vi "what_do_you_want.vi"() -> (0 "Next state":T1(ring), 1 "Leave":bool)   [LabVIEW 2014]
panel:
  in  "Cluster":T2
  # "You have pressed the cancel buttom.\nWhat do you want to do now?\n1.Choose seats again.\n2.Select another movie.\n3.Leave the movie booking system"
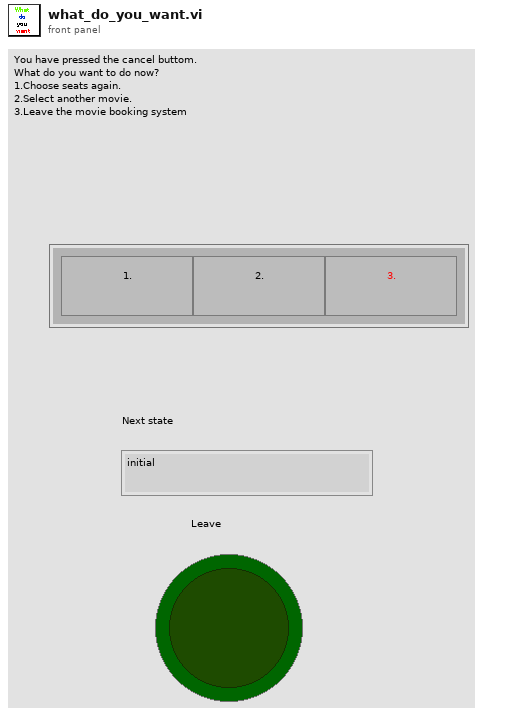
[diagram p1: front panel]
types:
  T1 = enum16{"initial", "start", "member?", "register?", "member login", "member register", "choose movie", "how many seat?", "check", "end"}
  T2 = cluster{"OK Button":bool, "OK Button 2":bool, "stop":bool}
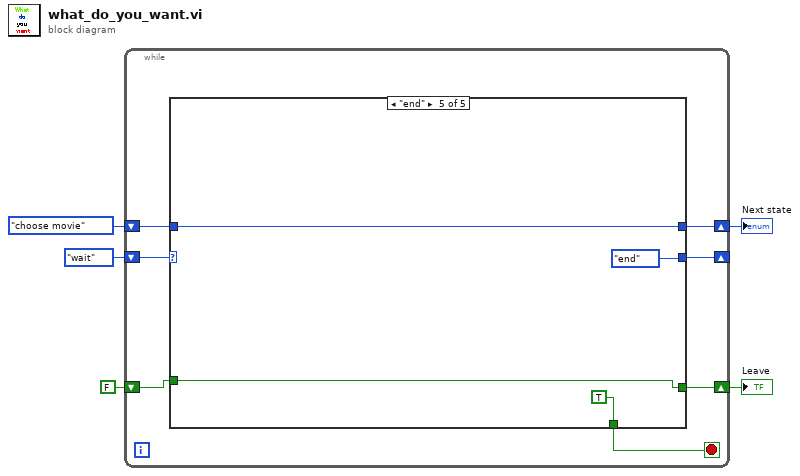
[diagram p0: block diagram]
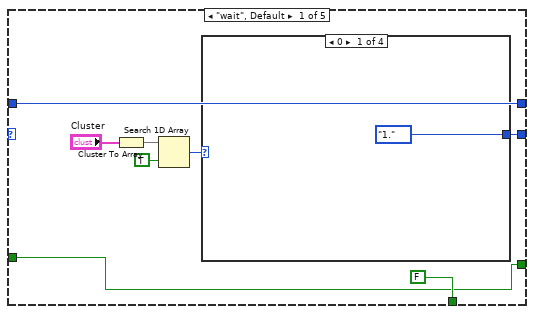
[diagram p2: hidden frame]
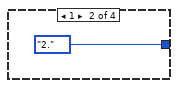
[diagram p3: hidden frame]
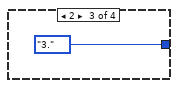
[diagram p4: hidden frame]
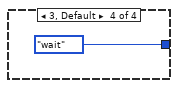
[diagram p5: hidden frame]
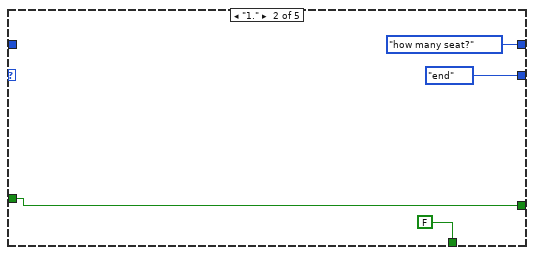
[diagram p6: hidden frame]
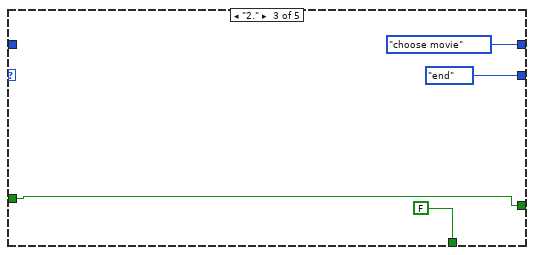
[diagram p7: hidden frame]
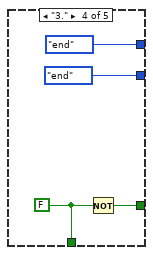
[diagram p8: hidden frame]
diagram:
  n1 = while {
    shift-right: [w11] -> _
    shift-left: enum16{"wait", "1.", "2.", "3.", "end"}."wait" -> [w12]
    shift-right: [w9] -> w3
    shift-left: T1."choose movie" -> [w10]
    shift-right: [w7] -> w2
    shift-left: FALSE -> [w6]
    stop <- w8 stop-if-true
    n2 = case shown="\"end\"" w12 {
      tunnel: [w16 enum16{"wait", "1.", "2.", "3.", "end"}."end" enum16{"wait", "1.", "2.", "3.", "end"}."end" enum16{"wait", "1.", "2.", "3.", "end"}."end" enum16{"wait", "1.", "2.", "3.", "end"}."end"] -> w11
      tunnel: [w15 T1."how many seat?" T1."choose movie" T1."end" w39] -> w9
      tunnel: w10 -> [w15 _ _ _ w39]
      tunnel: [FALSE FALSE FALSE w34 TRUE] -> w8
      tunnel: [w13 w25 w29 w33 w37] -> w7
      tunnel: w6 -> [w13 w25 w29 _ w37]
      frame "wait", Default {
        n3 = Cluster To Array(cluster="Cluster") -> (array=w19:bool[])
        n4 = Search 1D Array(1D array=w19, element=TRUE) -> (index of element=w17:i32)  [unwired: 1 in]
        n5 = case shown="0" w17 {
          tunnel: [enum16{"wait", "1.", "2.", "3.", "end"}."1." enum16{"wait", "1.", "2.", "3.", "end"}."2." enum16{"wait", "1.", "2.", "3.", "end"}."3." enum16{"wait", "1.", "2.", "3.", "end"}."wait"] -> w16
          frame 0 {
          }
          frame 1 {
          }
          frame 2 {
          }
          frame 3, Default {
          }
        }
      }
      frame "1." {
      }
      frame "2." {
      }
      frame "3." {
        w34 = FALSE
        n6 = Not(x=w34) -> (.not. x?=w33:bool)
      }
      frame "end" {
      }
    }
  }
  "Next state" <- w3
  "Leave" <- w2
